vi "main.vi"() -> ()   [LabVIEW 2022 SP3]
uses:
  <vilib>/Analysis/3filter.llb/Filter Passband Type.ctl
  2b79367e-ae1a-4011-bdbe-a47505f87f81.vi
  <extravilib>/ChannelInstances/Stream-ref(Queue(u16))/Write With Abort.vi
  <extravilib>/ChannelInstances/Stream-ref(Queue(u16))/Read With Abort.vi
  <extravilib>/ChannelInstances/Stream-ref(Queue(u16))/Endpoint.vi
  <extravilib>/ChannelInstances/Stream-ref(Queue(u16))/EndpointRead.vi
  <extravilib>/ChannelInstances/Stream-ref(Queue(u16))/Instantiate.vi
  <extravilib>/ChannelInstances/Stream-ref(Queue(u16))/)Channel.vi
  <resource>/ChannelSupport/_ChannelSupport/WaitIfNeeded.vi
  <vilib>/Analysis/3filter.llb/Butterworth Filter (DBL).vi
  <vilib>/measure/madcrms.llb/Basic Averaged DC-RMS for 1 Chan.vi
  <vilib>/Analysis/NI_AALBase.lvlib
  <extravilib>/ChannelInstances/Stream-ref(Queue(u16)).lvlib
  <vilib>/measure/NI_MAPro.lvlib
  <vilib>/Utility/file.llb/Read Delimited Spreadsheet (I64).vi
  <vilib>/measure/maspectr.llb/FFT Power Spectrum and PSD for 1 Chan.vi
  <vilib>/Utility/file.llb/Write Delimited Spreadsheet (I64).vi
  <vilib>/Instr/_visa.llb/VISA Configure Serial Port (Instr).vi
panel:
  in  "exert scan mode":bool=TRUE caption="模式"
  in  "exert threshold":dbl=250.0 caption="阈值"
  out "exert":bool caption="用力"
  in  "EMG waveform queue max length":i32=4096 caption="EMG 波形长度"
  out "stop light":bool
  in  "replay":bool
  in  "stop":bool
  out "EMG RMS value":dbl caption="EMG 均方根"
  out "EMG file length":i32 caption="EMG 文件长度"
  out "EMG filter progress":u8(slide) caption="滤波进度" scale=0.0..100.0
  out "EMG waveform length":i32 caption="当前长度"
  out "EMG value":u16 caption="补偿后值"
  out "EMG raw value":i32 caption="原始信号值"
  out "EMG enable flag":bool
  in  "选项卡控件":enum32{"默认采集页面", "滤波器", "功率谱", "回放"}(tab)
  out "EMG waveform":u16(graph)
  out "EMG raw waveform":dbl[](graph) caption="EMG 原始波形"
  out "EMG filtered waveform":u16[](graph) caption="EMG 滤波后波形"
  out "EMG PSD":cluster{"f0":dbl, "df":dbl, "magnitude":dbl[]}(graph) caption="EMG 功率谱"
  out "EMG replay":i64[][](graph)
  in  "EMG enable switch":bool
  in  "sampling freq":dbl=2014.0 caption="采样频率:fs" format="%0.2f"
  in  "EMG signal compensation":i32 caption="EMG 信号补偿值"
  in  "VISA resource name":refnum<visa-resource-name> caption="VISA资源名称"
  # "EMG 信号采集系统"
  # "A"
  # "B"
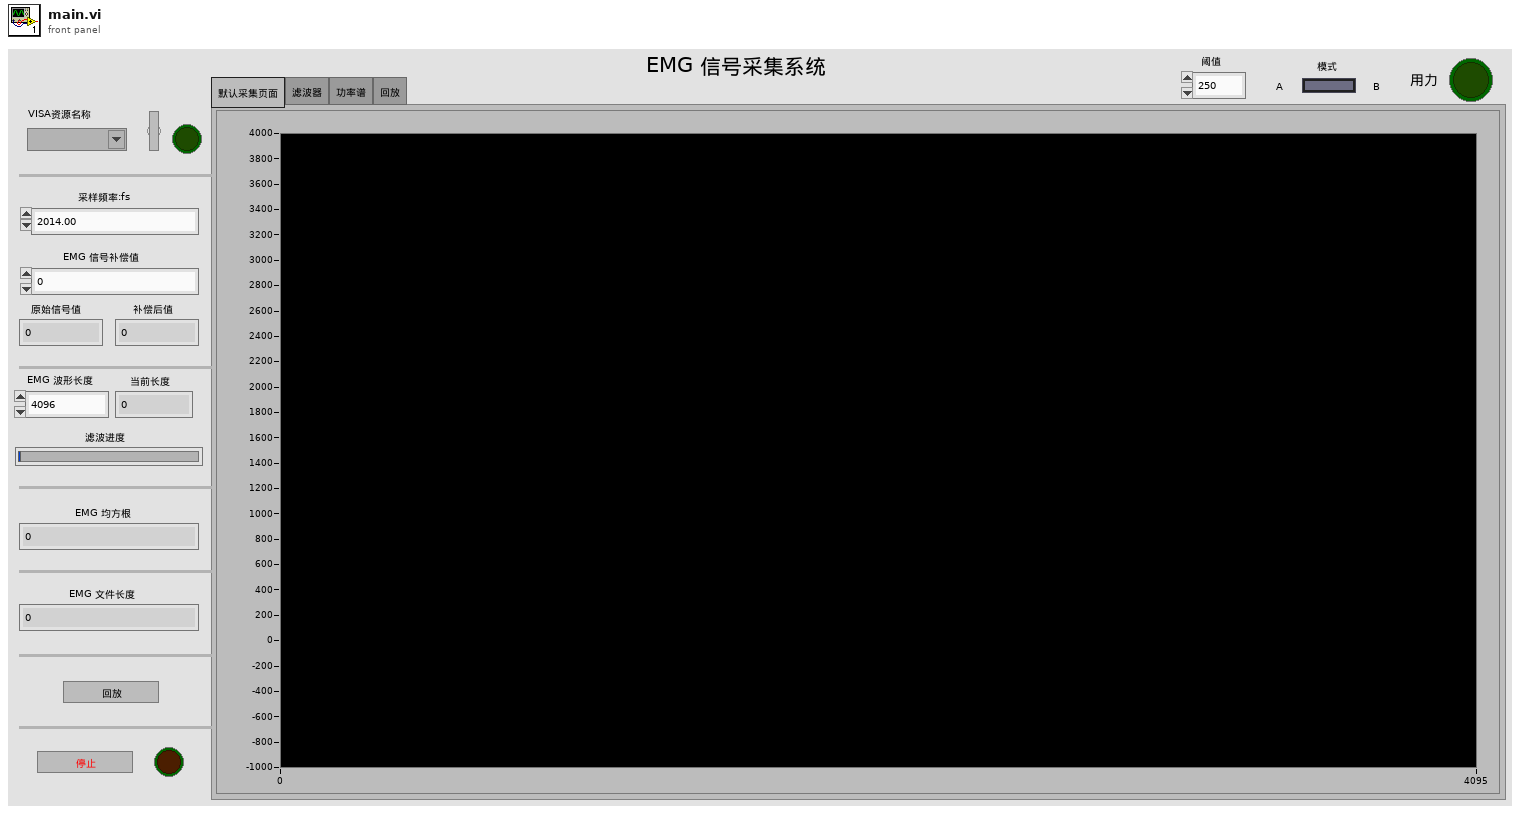
[diagram p1: front panel]
types:
  T1 = typedef "NI_AALBase.lvlib/Filter Passband Type.ctl" = enum32{"Lowpass", "Highpass", "Bandpass", "Bandstop"}
  T2 = typedef "Stream-ref(Queue(u16)).lvlib/)Channel.ctl" = refnum<queue>
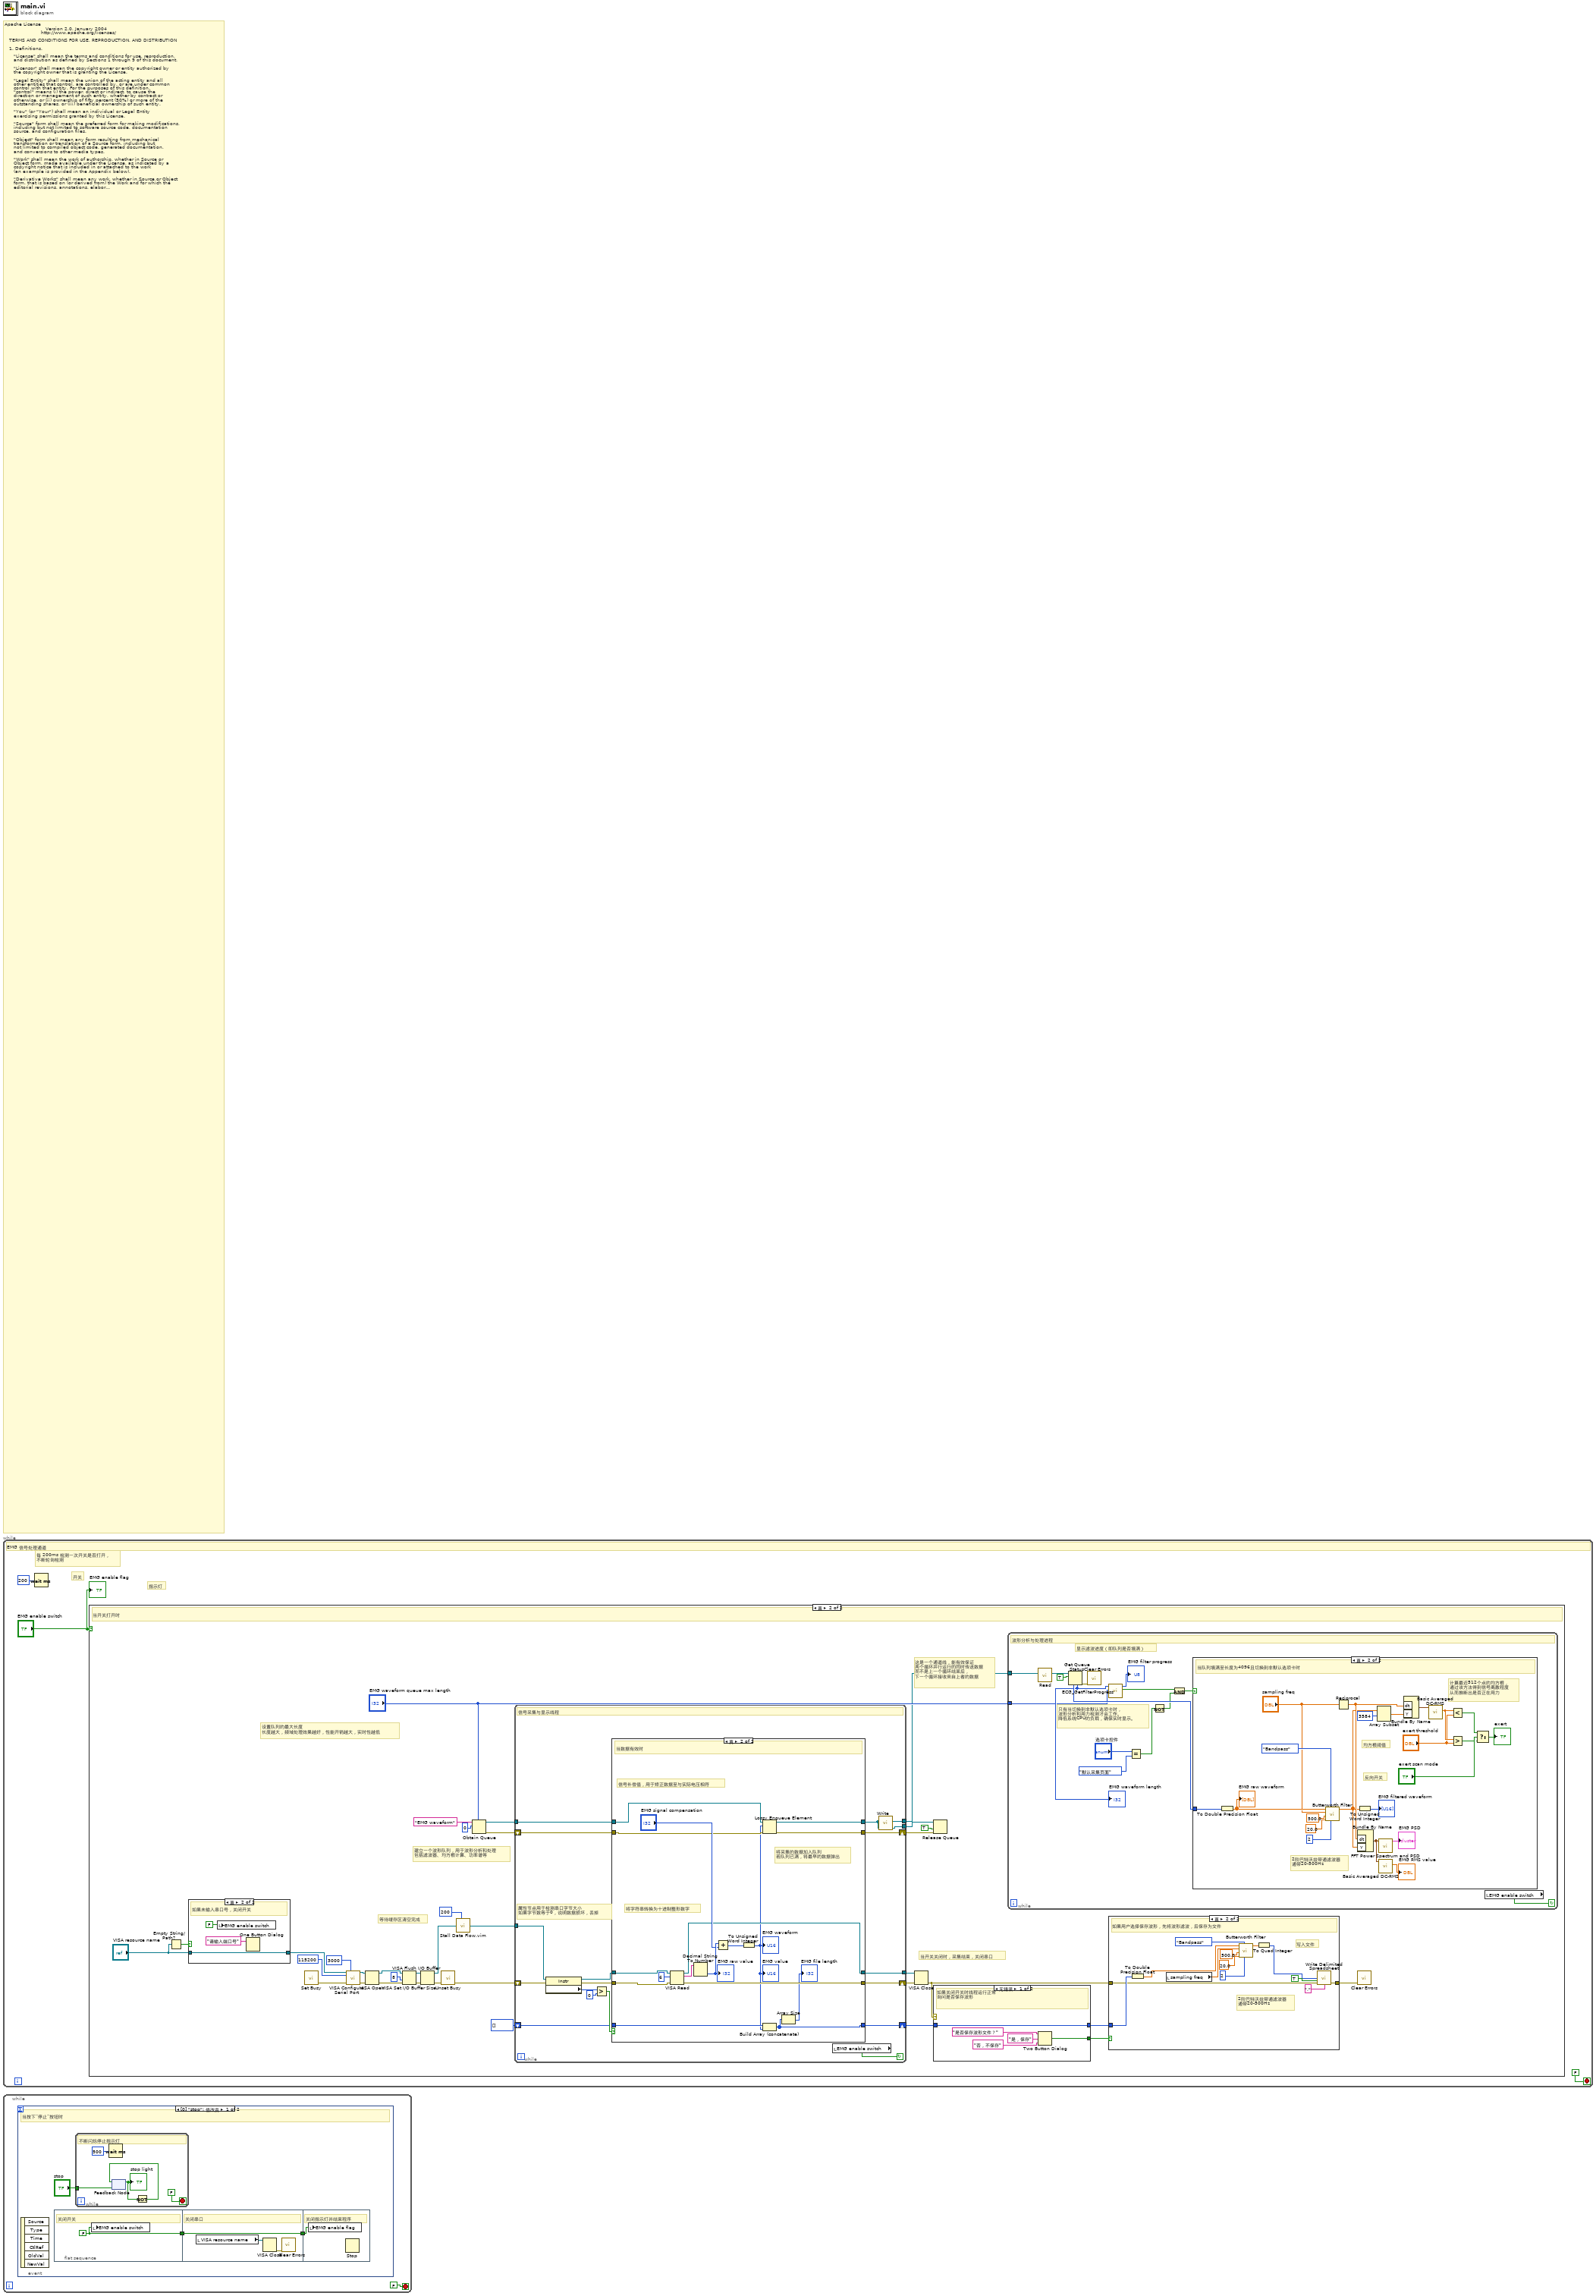
[diagram p0: block diagram]
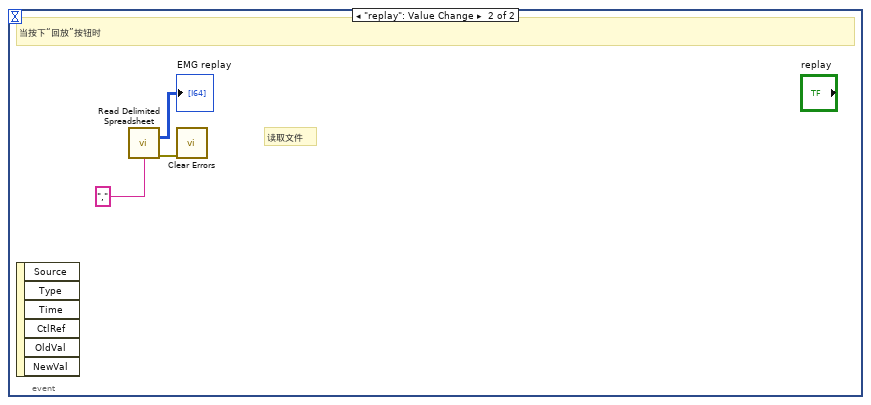
[diagram p2: hidden frame]
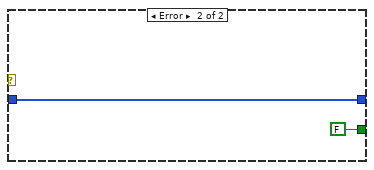
[diagram p5: hidden frame]
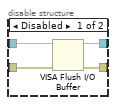
[diagram p9: hidden frame]
diagram:
  # "Apache License\n                           Version 2.0, January 2004\n                        http://www.apache.org/licenses/\n\n   TERMS AND CONDITIONS FOR USE, REPRODUCTION, AND DISTRIBUTION\n\n   1. Definitions.\n\n      \"License\" shall mean the terms and conditions for use, reproduction,\n      and distribution as defined by Sections 1 through 9 of this document.\n\n      \"Licensor\" shall mean the copyright owner or entity authorized by\n      the copyright owner that is granting the License.\n\n      \"Legal Entity\" shall mean the union of the acting entity and all\n      other entities that control, are controlled by, or are under common\n      control with that entity. For the purposes of this definition,\n      \"control\" means (i) the power, direct or indirect, to cause the\n      direction or management of such entity, whether by contract or\n      otherwise, or (ii) ownership of fifty percent (50%) or more of the\n      outstanding shares, or (iii) beneficial ownership of such entity.\n\n      \"You\" (or \"Your\") shall mean an individual or Legal Entity\n      exercising permissions granted by this License.\n\n      \"Source\" form shall mean the preferred form for making modifications,\n      including but not limited to software source code, documentation\n      source, and configuration files.\n\n      \"Object\" form shall mean any form resulting from mechanical\n      transformation or translation of a Source form, including but\n      not limited to compiled object code, generated documentation,\n      and conversions to other media types.\n\n      \"Work\" shall mean the work of authorship, whether in Source or\n      Object form, made available under the License, as indicated by a\n      copyright notice that is included in or attached to the work\n      (an example is provided in the Appendix below).\n\n      \"Derivative Works\" shall mean any work, whether in Source or Object\n      form, that is based on (or derived from) the Work and for which the\n      editorial revisions, annotations, elaborations, or other modifications\n      represent, as a whole, an original work of authorship. For the purposes\n      of this License, Derivative Works shall not include works that remain\n      separable from, or merely link (or bind by name) to the interfaces of,\n      the Work and Derivative Works thereof.\n\n      \"Contribution\" shall mean any work of authorship, including\n      the original version of the Work and any modifications or additions\n      to that Work or Derivative Works thereof, that is intentionally\n      submitted to Licensor for inclusion in the Work by the copyright owner\n      or by an individual or Legal Entity authorized to submit on behalf of\n      the copyright owner. For the purposes of this definition, \"submitted\"\n      means any form of electronic, verbal, or written communication sent\n      to the Licensor or its representatives, including but not limited to\n      communication on electronic mailing lists, source code control systems,\n      and issue tracking systems that are managed by, or on behalf of, the\n      Licensor for the purpose of discussing and improving the Work, but\n      excluding communication that is conspicuously marked or otherwise\n      designated in writing by the copyright owner as \"Not a Contribution.\"\n\n      \"Contributor\" shall mean Licensor and any individual or Legal Entity\n      on behalf of whom a Contribution has been received by Licensor and\n      subsequently incorporated within the Work.\n\n   2. Grant of Copyright License. Subject to the terms and conditions of\n      this License, each Contributor hereby grants to You a perpetual,\n      worldwide, non-exclusive, no-charge, royalty-free, irrevocable\n      copyright license to reproduce, prepare Derivative Works of,\n      publicly display, publicly perform, sublicense, and distribute the\n      Work and such Derivative Works in Source or Object form.\n\n   3. Grant of Patent License. Subject to the terms and conditions of\n      this License, each Contributor hereby grants to You a perpetual,\n      worldwide, non-exclusive, no-charge, royalty-free, irrevocable\n      (except as stated in this section) patent license to make, have made,\n      use, offer to sell, sell, import, and otherwise transfer the Work,\n      where such license applies only to those patent claims licensable\n      by such Contributor that are necessarily infringed by their\n      Contribution(s) alone or by combination of their Contribution(s)\n      with the Work to which such Contribution(s) was submitted. If You\n      institute patent litigation against any entity (including a\n      cross-claim or counterclaim in a lawsuit) alleging that the Work\n      or a Contribution incorporated within the Work constitutes direct\n      or contributory patent infringement, then any patent licenses\n      granted to You under this License for that Work shall terminate\n      as of the date such litigation is filed.\n\n   4. Redistribution. You may reproduce and distribute copies of the\n      Work or Derivative Works thereof in any medium, with or without\n      modifications, and in Source or Object form, provided that You\n      meet the following conditions:\n\n      (a) You must give any other recipients of the Work or\n          Derivative Works a copy of this License; and\n\n      (b) You must cause any modified files to carry prominent notices\n          stating that You changed the files; and\n\n      (c) You must retain, in the Source form of any Derivative Works\n          that You distribute, all copyright, patent, trademark, and\n          attribution notices from the Source form of the Work,\n          excluding those notices that do not pertain to any part of\n          the Derivative Works; and\n\n      (d) If the Work includes a \"NOTICE\" text file as part of its\n          distribution, then any Derivative Works that You distribute must\n          include a readable copy of the attribution notices contained\n          within such NOTICE file, excluding those notices that do not\n          pertain to any part of the Derivative Works, in at least one\n          of the following places: within a NOTICE text file distributed\n          as part of the Derivative Works; within the Source form or\n          documentation, if provided along with the Derivative Works; or,\n          within a display generated by the Derivative Works, if and\n          wherever such third-party notices normally appear. The contents\n          of the NOTICE file are for informational purposes only and\n          do not modify the License. You may add Your own attribution\n          notices within Derivative Works that You distribute, alongside\n          or as an addendum to the NOTICE text from the Work, provided\n          that such additional attribution notices cannot be construed\n          as modifying the License.\n\n      You may add Your own copyright statement to Your modifications and\n      may provide additional or different license terms and conditions\n      for use, reproduction, or distribution of Your modifications, or\n      for any such Derivative Works as a whole, provided Your use,\n      reproduction, and distribution of the Work otherwise complies with\n      the conditions stated in this License.\n\n   5. Submission of Contributions. Unless You explicitly state otherwise,\n      any Contribution intentionally submitted for inclusion in the Work\n      by You to the Licensor shall be under the terms and conditions of\n      this License, without any additional terms or conditions.\n      Notwithstanding the above, nothing herein shall supersede or modify\n      the terms of any separate license agreement you may have executed\n      with Licensor regarding such Contributions.\n\n   6. Trademarks. This License does not grant permission to use the trade\n      names, trademarks, service marks, or product names of the Licensor,\n      except as required for reasonable and customary use in describing the\n      origin of the Work and reproducing the content of the NOTICE file.\n\n   7. Disclaimer of Warranty. Unless required by applicable law or\n      agreed to in writing, Licensor provides the Work (and each\n      Contributor provides its Contributions) on an \"AS IS\" BASIS,\n      WITHOUT WARRANTIES OR CONDITIONS OF ANY KIND, either express or\n      implied, including, without limitation, any warranties or conditions\n      of TITLE, NON-INFRINGEMENT, MERCHANTABILITY, or FITNESS FOR A\n      PARTICULAR PURPOSE. You are solely responsible for determining the\n      appropriateness of using or redistributing the Work and assume any\n      risks associated with Your exercise of permissions under this License.\n\n   8. Limitation of Liability. In no event and under no legal theory,\n      whether in tort (including negligence), contract, or otherwise,\n      unless required by applicable law (such as deliberate and grossly\n      negligent acts) or agreed to in writing, shall any Contributor be\n      liable to You for damages, including any direct, indirect, special,\n      incidental, or consequential damages of any character arising as a\n      result of this License or out of the use or inability to use the\n      Work (including but not limited to damages for loss of goodwill,\n      work stoppage, computer failure or malfunction, or any and all\n      other commercial damages or losses), even if such Contributor\n      has been advised of the possibility of such damages.\n\n   9. Accepting Warranty or Additional Liability. While redistributing\n      the Work or Derivative Works thereof, You may choose to offer,\n      and charge a fee for, acceptance of support, warranty, indemnity,\n      or other liability obligations and/or rights consistent with this\n      License. However, in accepting such obligations, You may act only\n      on Your own behalf and on Your sole responsibility, not on behalf\n      of any other Contributor, and only if You agree to indemnify,\n      defend, and hold each Contributor harmless for any liability\n      incurred by, or claims asserted against, such Contributor by reason\n      of your accepting any such warranty or additional liability.\n\n   END OF TERMS AND CONDITIONS\n\n   APPENDIX: How to apply the Apache License to your work.\n\n      To apply the Apache License to your work, attach the following\n      boilerplate notice, with the fields enclosed by brackets \"[]\"\n      replaced with your own identifying information. (Don't include\n      the brackets!)  The text should be enclosed in the appropriate\n      comment syntax for the file format. We also recommend that a\n      file or class name and description of purpose be included on the\n      same \"printed page\" as the copyright notice for easier\n      identification within third-party archives.\n\n   Copyright [yyyy] [name of copyright owner]\n\n   Licensed under the Apache License, Version 2.0 (the \"License\");\n   you may not use this file except in compliance with the License.\n   You may obtain a copy of the License at\n\n       http://www.apache.org/licenses/LICENSE-2.0\n\n   Unless required by applicable law or agreed to in writing, software\n   distributed under the License is distributed on an \"AS IS\" BASIS,\n   WITHOUT WARRANTIES OR CONDITIONS OF ANY KIND, either express or implied.\n   See the License for the specific language governing permissions and\n   limitations under the License."
  n1 = while {
    stop <- FALSE stop-if-true
    # "开关"
    # "指示灯"
    # "每 200ms 检测一次开关是否打开，\n不断轮询检测"
    # "EMG 信号处理通道"
    n2 = Wait (ms)(milliseconds to wait=u32 200 ("等待时间（毫秒）")) -> ()  [unwired: 1 out]
    n3 = case shown="真" "EMG enable switch" {
      frame False {
      }
      frame True {
        # "这是一个通道线，能有效保证\n两个循环并行运行的同时传送数据\n而不是上一个循环结束后，\n下一个循环接收来自上者的数据"
        # "当开关关闭时，采集结束，关闭串口"
        # "设置队列的最大长度\n长度越大，频域处理效果越好，性能开销越大，实时性越低"
        # "建立一个波形队列，用于波形分析和处理\n包括滤波器、均方根计算、功率谱等"
        # "等待缓存区清空完成"
        # "当开关打开时"
        n4 = Empty String/Path?(string/path="VISA resource name") -> (empty?=w6:bool)
        n5 = case shown="真" w6 {
          tunnel: [w39 w40] -> w5
          tunnel: "VISA resource name" -> [w39 w40]
          frame False {
          }
          frame True {
            # "如果未输入串口号，关闭开关"
            n6 = local write "EMG enable switch"(FALSE ("EMG enable switch")) -> ()
            n7 = One Button Dialog(message="请输入端口号" ("消息")) -> ()  [unwired: 1 in, 1 out]
          }
        }
        n8 = call <vilib>:"Set Busy.vi"() -> ("error out"=w11:errorcluster)  [unwired: 10 in, 1 out]
        n9 = call-poly "VISA Configure Serial Port"("VISA resource name"=w5, "timeout (10sec)"=u32 3000, "baud rate (9600)"=u32 115200, "error in (no error)"=w11) -> ("VISA resource name out"=w33:refnum<visa-resource-name>, "error out"=w34:errorcluster)  [unwired: 10 in]
        n10 = VISA Open(error in (no error)=w34, VISA resource name=w33) -> (VISA resource name=w37:refnum<visa-resource-name>, error out=w36:errorcluster)  [unwired: 3 in]
        n11 = VISA Set I/O Buffer Size(VISA resource name=w37, size (4096)=u32 8 ("大小(4096)"), error in (no error)=w36) -> (VISA resource name out=w31:refnum<visa-resource-name>, error out=w32:errorcluster)  [unwired: 1 in]
        n12 = VISA Flush I/O Buffer(VISA resource name=w31, error in (no error)=w32) -> (VISA resource name out=w27:refnum<visa-resource-name>, error out=w10:errorcluster)  [unwired: 1 in]
        n13 = call <vilib>:"Unset Busy.vi"("error in (no error)"=w10) -> ("error out"=w9:errorcluster)  [unwired: 10 in]
        n14 = call "Stall Data Flow.vim"("value in"=w27, "milliseconds to wait"=u32 200) -> ("value out"=w26:refnum<visa-resource-name>)  [unwired: 1 out]
        n15 = Obtain Queue(max queue size (-1, unlimited)="EMG waveform queue max length", name (unnamed)="EMG waveform" ("名称（未命名）"), element data type=u16 0) -> (queue out=w22:refnum<queue>, error out=w21:errorcluster)  [unwired: 2 in, 1 out]
        n16 = while {
          tunnel: w26 -> [w117]
          tunnel: [w110] -> w24
          tunnel: w22 -> [w108]
          tunnel: [w106] -> w19
          tunnel: [w103] -> w16
          shift-right: [w101] -> w12
          shift-left: u16[] [] -> [w102]
          shift-right: [w105] -> w18
          shift-left: w21 -> [w107]
          shift-right: [w109] -> w23
          shift-left: w9 -> [w116]
          stop <- w104 continue-if-true
          # "属性节点用于检测串口字节大小\n如果字节数等于0，说明数据损坏，丢掉"
          # "信号采集与显示线程"
          n17 = property class="Instr"(reference=w117, error in=w116) -> (reference out=w113:refnum<visa-resource-name>, error out=w112:errorcluster, "Serial Settings:Number of Bytes at Serial Port"=w114:u32)
          n18 = Greater?(x=w114, y=u32 0) -> (0:w111:bool)
          n19 = case shown="真" w111 {
            tunnel: w113 -> [w124 w147]
            tunnel: w112 -> [w123 w146]
            tunnel: [w122 w140] -> w110
            tunnel: [w121 w139] -> w109
            tunnel: w108 -> [w120 w138]
            tunnel: w107 -> [w119 w137]
            tunnel: [w120 w136] -> w106
            tunnel: [w119 w135] -> w105
            tunnel: w102 -> [w118 w134]
            tunnel: [w118 w133] -> w101
            frame False {
              n20 = disable-structure shown="启用" {
                disable-tunnel: w124 -> [w128 w130]
                disable-tunnel: w123 -> [w127 w129]
                disable-tunnel: [w126 w130] -> w122
                disable-tunnel: [w125 w129] -> w121
                frame Disabled {
                  n21 = VISA Flush I/O Buffer(VISA resource name=w128, error in (no error)=w127) -> (VISA resource name out=w126:refnum<visa-resource-name>, error out=w125:errorcluster)  [unwired: 1 in]
                }
                frame Enabled {
                }
              }
            }
            frame True {
              # "将采集的数据加入队列\n若队列已满，将最早的数据弹出"
              # "将字符串转换为十进制整形数字"
              # "信号补偿值，用于矫正数据至与实际电压相符"
              # "当数据有效时"
              n22 = VISA Read(VISA resource name=w147, byte count=u32 6 ("字节总数"), error in (no error)=w146) -> (VISA resource name out=w140:refnum<visa-resource-name>, read buffer=w144:string, error out=w139:errorcluster)  [unwired: 1 out]
              n23 = Decimal String To Number(string=w144) -> (number=w143:i32)  [unwired: 2 in, 1 out]
              "EMG raw value" <- w143
              n24 = Add(x=w143, y="EMG signal compensation") -> (x+y=w141:i32)
              n25 = To Unsigned Word Integer(number=w141) -> (unsigned 16bit integer=w131:u16)
              "EMG waveform" <- w131
              "EMG value" <- w131
              n26 = Lossy Enqueue Element(queue=w138, element=w131, error in (no error)=w137) -> (queue out=w136:refnum<queue>, error out=w135:errorcluster)  [unwired: 2 out]
              n27 = Build Array (concatenate)(w134, w131) -> (w133:u16[])
              n28 = Array Size(array=w133) -> (size(s)=→"EMG file length":i32)
            }
          }
          n29 = local read "EMG enable switch"() -> (w104:bool)
          n30 = call <extravilib>:"Write.vi"("element"=w106) -> ("channel"=w103:T2)  [unwired: 8 in, 2 out]
        }
        n31 = VISA Close(VISA resource name=w24, error in (no error)=w23) -> (error out=w7:errorcluster)
        n32 = Release Queue(queue=w19, force destroy? (F)=TRUE ("强制销毁？(F)"), error in (no error)=w18) -> ()  [unwired: 3 out]
        n33 = case shown="无错误" w7 {
          tunnel: [w47 FALSE ("T button?")] -> w14
          tunnel: [w46 w48] -> w13
          tunnel: w12 -> [w46 w48]
          frame No Error {
            # "如果关闭开关时线程运行正常\n询问是否保存波形"
            n34 = Two Button Dialog(message="是否保存波形文件？" ("消息"), 1:"否，不保存" ("F按钮名称（“取消”）"), 2:"是，保存" ("T按钮名称（“确定”）")) -> (T button?=w47:bool)
          }
          frame Error {
          }
        }
        n35 = while {
          tunnel: "EMG waveform queue max length" -> [w54]
          tunnel: w16 -> [w63]
          stop <- w61 continue-if-true
          # "只有当切换到非默认选项卡时，\n波形分析和用力检测才会工作。\n降低系统CPU的负载，确保实时显示。"
          # "显示滤波进度（即队列是否填满）"
          # "波形分析与处理进程"
          n36 = call <extravilib>:"Read.vi"("channel"=w63) -> ("element"=w62:refnum<queue>)  [unwired: 6 in, 4 out]
          n37 = Get Queue Status(queue=w62, return elements? (F)=TRUE ("返回元素？(F)")) -> (error out=w51:errorcluster, # elements in queue=w55:i32, elements=w64:u16[])  [unwired: 1 in, 5 out]
          "EMG waveform length" <- w55
          n38 = call <vilib>:"Clear Errors.vi"("error in (no error)"=w51) -> ()  [unwired: 5 in, 2 out]
          n39 = call "ECG_GetFilterProgress.vi"("target length"=w54, "current length"=w55) -> ("done"=w53:bool, "progress"=→"EMG filter progress":u8)  [unwired: 7 in, 1 out]
          n40 = Equal?(x="选项卡控件", y=enum32{"默认采集页面", "滤波器", "功率谱", "回放"}."默认采集页面") -> (x = y?=w57:bool)
          n41 = Not(x=w57) -> (.not. x?=w56:bool)
          n42 = And(x=w53, y=w56) -> (x .and. y?=w58:bool)
          n43 = case shown="真" w58 {
            tunnel: w64 -> [_ w86]
            frame False {
            }
            frame True {
              # "2阶巴特沃兹带通滤波器\n通带20-500Hz"
              # "均方根阈值"
              # "反向开关"
              # "计算最近512个点的均方根，\n通过该方法得到信号离散程度\n从而推断出是否正在用力"
              # "当队列填满至长度为4096且切换到非默认选项卡时"
              n44 = To Double Precision Float(number=w86) -> (double precision float=w80:dbl[])
              "EMG raw waveform" <- w80
              n45 = call-poly <vilib>:"Butterworth Filter.vi"("order"=2, "filter type"=Filter_Passband_Type."Bandpass", "low cutoff freq: fl"=20.0, "high cutoff freq: fh"=500.0, "sampling freq: fs"="sampling freq", "X"=w80) -> ("Filtered X"=w65:dbl[])  [unwired: 2 in, 1 out]
              n46 = Reciprocal(x="sampling freq") -> (1/x=w74:dbl)
              n47 = Bundle By Name("dt"=w74, "Y"=w65) -> (w77:waveform(dbl))  [unwired: 1 in]
              n48 = To Unsigned Word Integer(number=w65) -> (unsigned 16bit integer=→"EMG filtered waveform":u16[])
              n49 = Array Subset(array=w65, index=3584 ("索引")) -> (w75:dbl[])  [unwired: 1 in]
              n50 = call-poly <vilib>:"FFT Power Spectrum and PSD.vi"("time signal"=w77) -> ("Power Spectrum / PSD"=→"EMG PSD":cluster{"f0":dbl, "df":dbl, "magnitude":dbl[]})  [unwired: 7 in, 3 out]
              n51 = call-poly <vilib>:"Basic Averaged DC-RMS.vi"("signal in"=w77) -> ("RMS value"=→"EMG RMS value":dbl)  [unwired: 7 in, 3 out]
              n52 = Bundle By Name("dt"=w74, "Y"=w75) -> (w73:waveform(dbl))  [unwired: 1 in]
              n53 = call-poly <vilib>:"Basic Averaged DC-RMS.vi"("signal in"=w73) -> ("RMS value"=w71:dbl)  [unwired: 7 in, 3 out]
              n54 = Less?(x=w71, y="exert threshold") -> (x < y?=w69:bool)
              n55 = Greater?(x=w71, y="exert threshold") -> (0:w68:bool)
              n56 = Select(t=w69, s="exert scan mode", f=w68) -> (s? t:f=→"exert":bool)
            }
          }
          n57 = local read "EMG enable switch"() -> (w61:bool)
        }
        n58 = case shown="真" w14 {
          tunnel: w13 -> [_ w94]
          tunnel: w7 -> [w87 w90]
          tunnel: [w87 w89] -> w8
          frame False {
          }
          frame True {
            # "写入文件"
            # "2阶巴特沃兹带通滤波器\n通带20-500Hz"
            # "如果用户选择保存波形，先将波形滤波，后保存为文件"
            n59 = To Double Precision Float(number=w94) -> (double precision float=w93:dbl[])
            n60 = local read "sampling freq"() -> (w92:dbl)
            n61 = call-poly <vilib>:"Butterworth Filter.vi"("order"=2, "filter type"=Filter_Passband_Type."Bandpass", "low cutoff freq: fl"=20.0, "high cutoff freq: fh"=500.0, "sampling freq: fs"=w92, "X"=w93) -> ("Filtered X"=w91:dbl[])  [unwired: 2 in, 1 out]
            n62 = To Quad Integer(1:w91) -> (0:w99:i64[])
            n63 = call-poly <vilib>:"Write Delimited Spreadsheet.vi"("1D data"=w99, "append to file? (new file:F)"=TRUE, "error in (no error)"=w90, "delimiter (\\t)"="," ("delimiter (\\t)")) -> ("error out"=w89:errorcluster)  [unwired: 10 in, 1 out]
          }
        }
        n64 = call <vilib>:"Clear Errors.vi"("error in (no error)"=w8) -> ()  [unwired: 5 in, 2 out]
      }
    }
    "EMG enable flag" <- "EMG enable switch"
  }
  n65 = while {
    stop <- FALSE stop-if-true
    n66 = event shown="[0] \"stop\": 值改变" {
      selector: _ -> [_ _]
      dyn-events: _ -> [_ _]
      timeout: _ -> [_ _]
      event "stop": Value Change {
        # "当按下”停止“按钮时"
        n67 = event-data() -> ()  [unwired: 1 in, 6 out]
        n68 = flat-sequence {
          tunnel: [w152] -> w149
          tunnel: [w153] -> w150
          tunnel: w149 -> [w153]
          tunnel: w150 -> [w156]
          frame #0 {
            w152 = FALSE ("EMG enable switch")
            # "关闭开关"
            n69 = local write "EMG enable switch"(w152) -> ()
          }
          frame #1 {
            # "关闭串口"
            n70 = local read "VISA resource name"() -> (w154:refnum<visa-resource-name>)
            n71 = VISA Close(VISA resource name=w154) -> (error out=w155:errorcluster)  [unwired: 1 in]
            n72 = call <vilib>:"Clear Errors.vi"("error in (no error)"=w155) -> ()  [unwired: 5 in, 2 out]
          }
          frame #2 {
            # "关闭指示灯并结束程序"
            n73 = local write "EMG enable flag"(w156) -> ()
            n74 = Stop() -> ()  [unwired: 1 in]
          }
        }
        n75 = while {
          tunnel: "stop" -> [w158]
          stop <- FALSE stop-if-true
          # "不断闪烁停止指示灯"
          n76 = Wait (ms)(milliseconds to wait=u32 500 ("等待时间（毫秒）")) -> ()  [unwired: 1 out]
          n77 = feedback #1(w158) -> (w159:bool)
          "stop light" <- w159
          n78 = Not(x=w159) -> (.not. x?=w160:bool)
          n79 = feedback-in #1(w160) -> ()
        }
      }
      event "replay": Value Change {
        # "读取文件"
        # "当按下“回放”按钮时"
        n80 = event-data() -> ()  [unwired: 1 in, 6 out]
        n81 = call-poly <vilib>:"Read Delimited Spreadsheet.vi"("delimiter (\\t)"="," ("delimiter (\\t)")) -> ("all rows"=→"EMG replay":i64[][], "error out"=w162:errorcluster)  [unwired: 9 in, 4 out]
        n82 = call <vilib>:"Clear Errors.vi"("error in (no error)"=w162) -> ()  [unwired: 5 in, 2 out]
      }
    }
  }
